vi "Set Port.vi"(8 "error in (no error)":errorcluster, 10 "Port":u16, 11 "URI in":refnum<class "URI.lvclass">) -> (0 "error out":errorcluster, 3 "URI out":refnum<class "URI.lvclass">)   [LabVIEW 2020, in "IO.lvlib" / "URI.lvclass"]
uses:
  URI.lvclass
  URI.lvclass/URI.ctl
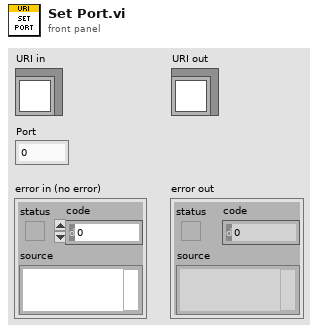
[diagram p1: front panel]
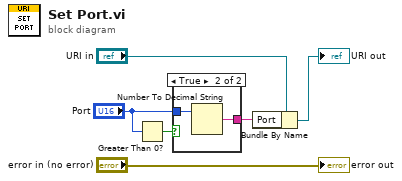
[diagram p0: block diagram]
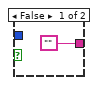
[diagram p2: hidden frame]
diagram:
  n1 = Greater Than 0?(x="Port") -> (x > 0?=w1:bool)
  n2 = case shown="True" w1 {
    tunnel: ["" w9] -> w5
    tunnel: "Port" -> [_ w8]
    frame False {
    }
    frame True {
      n3 = Number To Decimal String(number=w8) -> (decimal integer string=w9:string)  [unwired: 1 in]
    }
  }
  n4 = Bundle By Name(cluster="URI in", "Port"=w5) -> (→"URI out":refnum<class "URI.lvclass">)
  "error out" <- "error in (no error)"
